vi "Start Heartbeat Producer.vi"(8 "error in":errorcluster, 10 "Interval":i32 format="%d ms", 11 "CANopen Master in":refnum<class "CANopen Master.lvclass">) -> (0 "error out":errorcluster, 3 "CANopen Master out":refnum<class "CANopen Master.lvclass">)   [LabVIEW 2024, in "CANopen Master.lvlib" / "CANopen Master.lvclass"]
uses:
  CANopen Master.lvclass
  CANopen Master.lvclass/CANopen Master.ctl
  Heartbeat Producer.vi
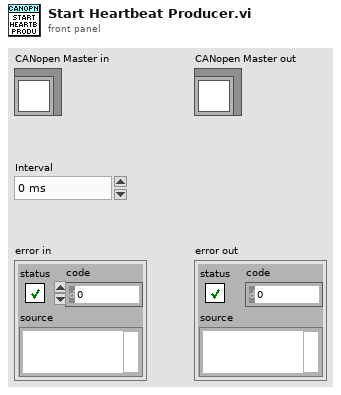
[diagram p1: front panel]
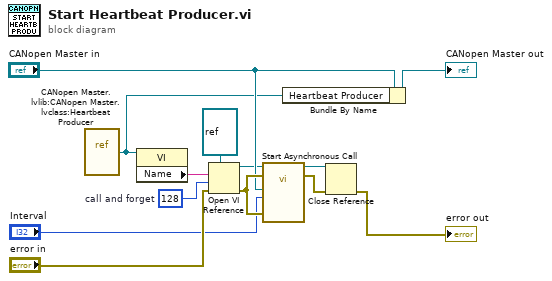
[diagram p0: block diagram]
diagram:
  w13 = 128  # call and forget
  n1 = vi-ref "CANopen Master.lvlib:CANopen Master.lvclass:Heartbeat Producer.vi"() -> (w2:refnum<vi>)
  n2 = property class="VI"(reference=w2) -> ("Name"=w10:string)  [unwired: 1 in, 2 out]
  n3 = Open VI Reference(type specifier VI Refnum (for type only)=refnum<vi> refnum, vi path=w10, options=w13, error in (no error)="error in") -> (vi reference=w4:refnum<vi>, error out=w11:errorcluster)  [unwired: 2 in]
  n4 = call-by-ref "Start Asynchronous Call"(reference=w4, error in=w11, "error in"=w11, "Interval"="Interval", "CANopen Master in"="CANopen Master in") -> (reference out=w5:refnum<vi>, error out=w12:errorcluster)  [unwired: 9 in]
  n5 = Bundle By Name(cluster="CANopen Master in", "Heartbeat Producer"=w2) -> (→"CANopen Master out":refnum<class "CANopen Master.lvclass">)
  n6 = Close Reference(reference=w5, error in (no error)=w12) -> (error out=→"error out":errorcluster)
